vi "CtrExtTrigAuger.vi"() -> ()   [LabVIEW 2014]
uses:
  FPGA state.ctl
  <vilib>/Platform/TimedLoop/XDataNode/timing_clust.ctl
  <vilib>/Platform/TimedLoop/XDataNode/nitl_modes.ctl
  <vilib>/Platform/TimedLoop/XDataNode/wakeup.ctl
  <vilib>/rvi/Emulation/niFpgaSctlEmulationGetInTimedLoop.vi
  <vilib>/rvi/Emulation/niFpgaEmulationReportErrorSimple.vi
  <vilib>/rvi/Emulation/niFpgaGetClockAttributes.vi
  <vilib>/rvi/Emulation/niFpgaCriticalErrorInLSC.vi
  <vilib>/rvi/eio/common/nirviEmuTemplateMethod_errors.vi
  <vilib>/rvi/Emulation/niFpgaProcessEmulError.vi
  <vilib>/rvi/interface/RandomDataEmulation/niFpgaRandomDataHandleErrors.vi
  <vilib>/Platform/TimedLoop/XDataNode/XDataNode.xnode
  <vilib>/eio/EIONode/EIONode.xnode
  <vilib>/rvi/DataTransferAndStorage/Container/XNode/niFpgaContainer.xnode
  <vilib>/rvi/interface/RandomDataEmulation/nirviRandomDataFpgaReadWriteTemplate.vi
  <vilib>/Platform/TimedLoop/XDataNode/XDNodeRunTimeDep.lvlib
panel:
  in  "Sample Count":u32
  in  "Sample Period":u32
  out "Overflow":bool
  in  "Trigger Mode":T1(ring)
  # "Acquisition can be controlled by external trigger\n(through PXI backplane or input connector)\nor by the FPGA 25 MHz Clock."
  # "ExtTrig AugerCounter"
  # "Each U64 FIFO element is a pair of U32 with\n28 bits data, 4 bit ID in most significant bits\nID 0-7 for data channels, 8 for clock and 9 for trig count\n\nOn trigger return sample count, delta T in first element,\nand counts since last trigger on the eight data channels\n(7 for Auger plus aux) in the next 4 elements\n\nOn overflow, set trigger mode to off and flush FIFO\nOFF mode clears overflow, also resests sample count"
  # "(40 ns/25 MHz)"
  # "(0 for free-run)"
  # "FPGA DMA-FIFO CANNOT be cleared by FPGA,\nonly by PC Host VI. Ctr Overflow will be on when\nFPGA-side FIFO is full!"
  # "Red for overflow\ngreen for normal"
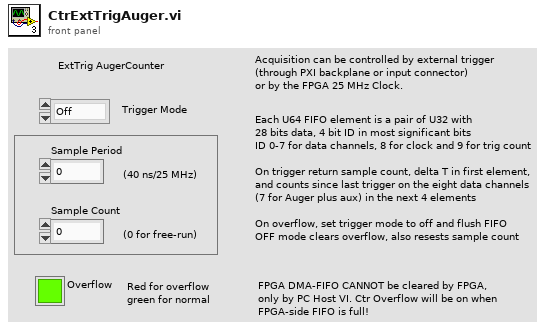
[diagram p1: front panel]
types:
  T1 = enum8{"Off", "PXI Trig0", "DIO-08 Trig", "Int Timer"}
  T2 = typedef "FPGA state.ctl" = enum8{"Wait", "Triggered", "Transfer 1", "Transfer 2", "Transfer 3", "Transfer 4", "Overflow"}
  T3 = typedef "XDNodeRunTimeDep.lvlib/timing_clust.ctl" = cluster{"Expected End [f-1]":u64, "Actual End [f-1]":u64, "Finished Late? [f-1]":bool, "Expected End [i-1]":u64, "Actual End [i-1]":u64, "Finished Late? [i-1]":bool, "Expected Start [i]":u64, "Actual Start [i]":u64, "Expected Start [f]":u64, "Actual Start [f]":u64, "Source Name":string, "Structure Name":string, "Period":i64, "Deadline":i64, "Offset":i64, "Start":i64, "Priority":i32, "Timeout":i32, "Mode":T4, "Wakeup Reason":T5, "Error":errorcluster, "Source Type":string, "Secondary Source Type":string, "Global End Time":u64, "Global Start Time":u64, "Frame Duration":u64, "Iteration Duration":u64, "Assigned CPU":i32, "I/O Scan Engine Mode":u32}
  T4 = typedef "XDNodeRunTimeDep.lvlib/nitl_modes.ctl" = enum32{"No Change", "Process missed periods, maintain original phase", "Discard missed periods, maintain original phase", "Process missed periods, ignore original phase", "Discard missed periods, ignore original phase"}
  T5 = typedef "XDNodeRunTimeDep.lvlib/wakeup.ctl" = enum32{"Normal", "Aborted", "Asynchronous wakeup", "Timing source error", "Timed loop error", "Timeout"}
  T6 = enum8{"Off", "PXI Trig0", "DIO-08 Trig", "Clocked"}
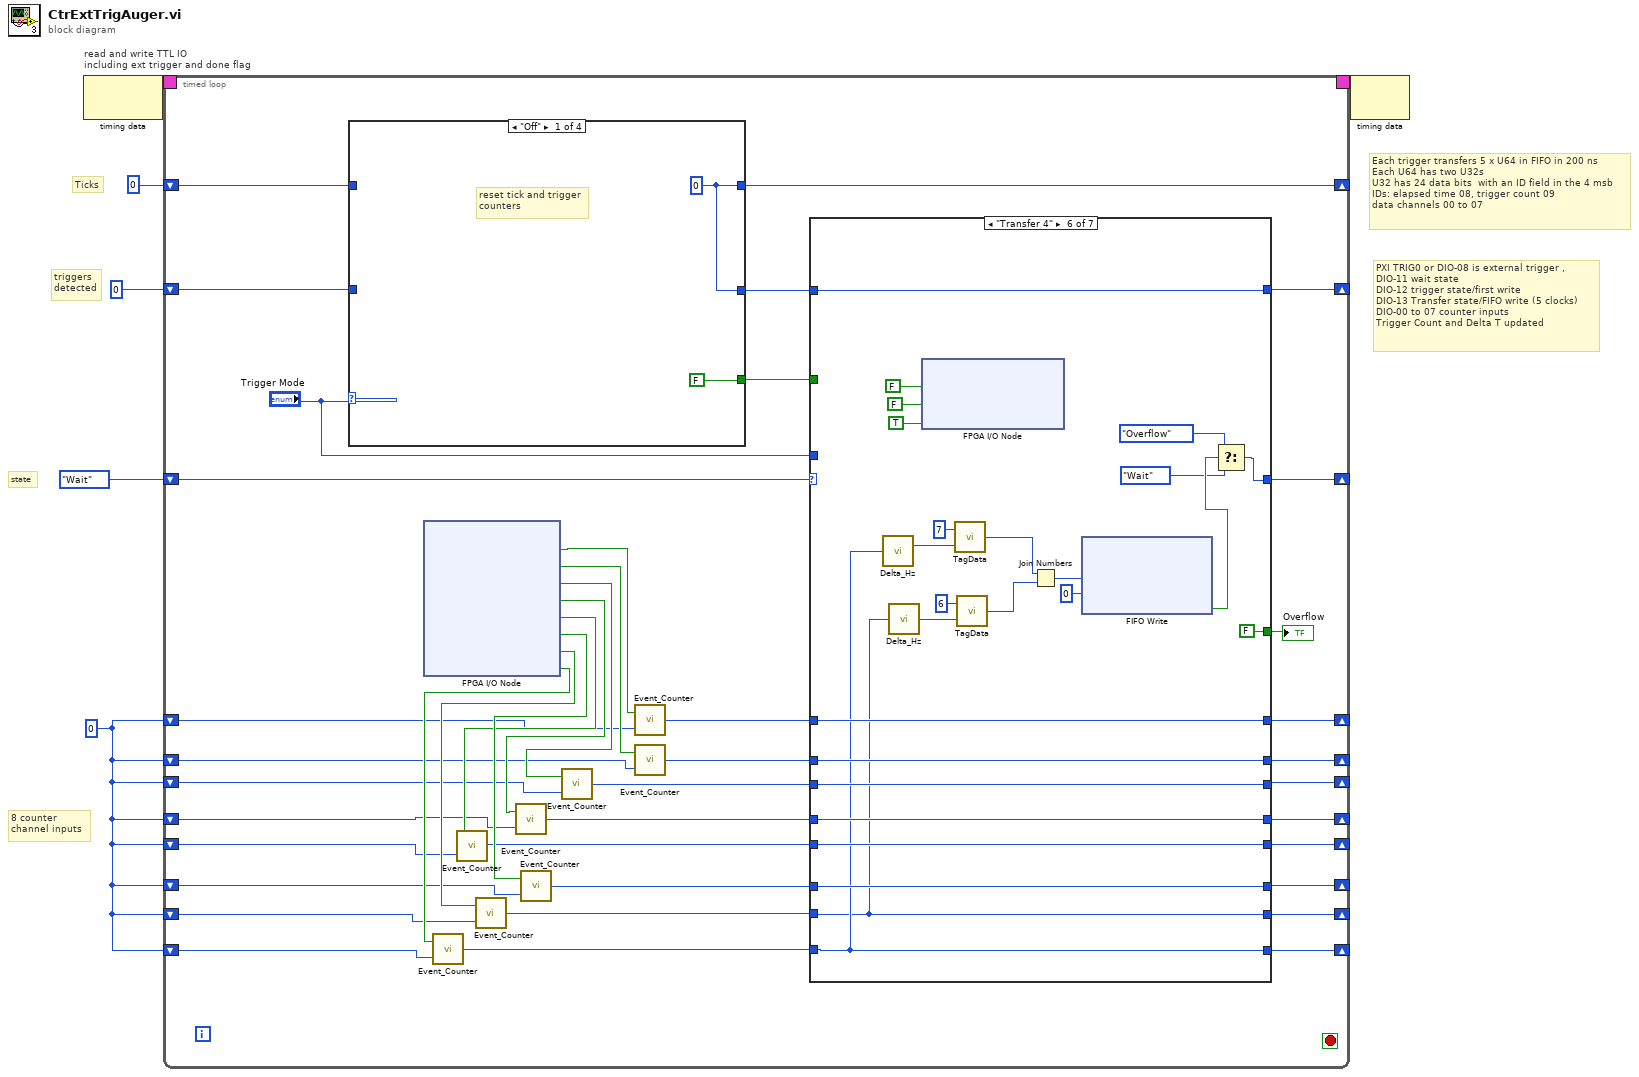
[diagram p0: block diagram]
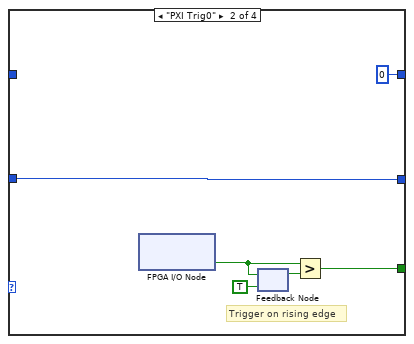
[diagram p2: hidden frame]
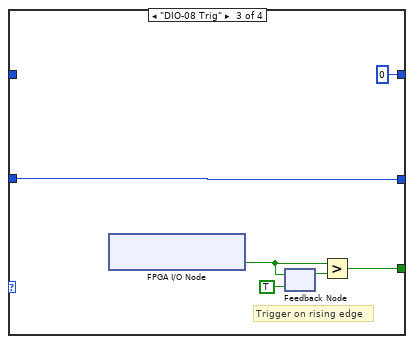
[diagram p3: hidden frame]
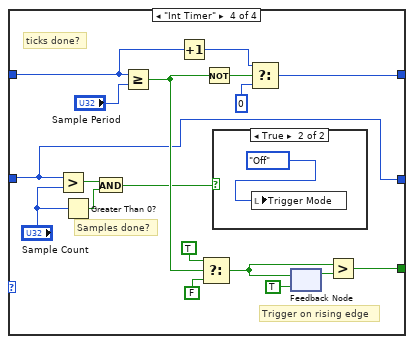
[diagram p4: hidden frame]
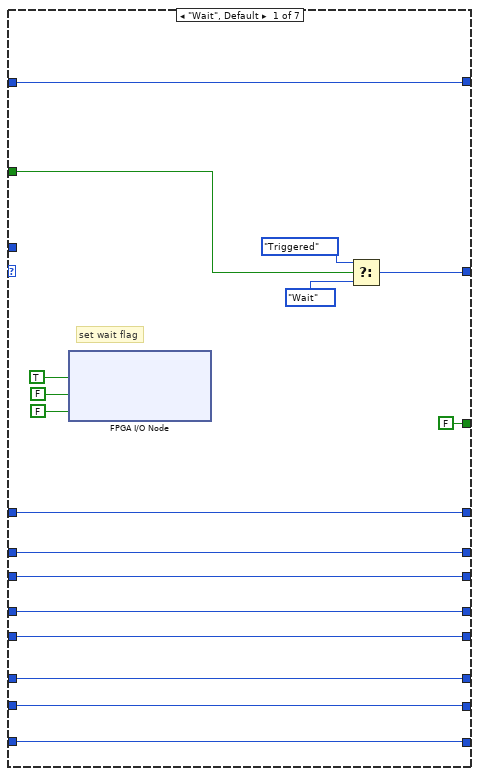
[diagram p6: hidden frame]
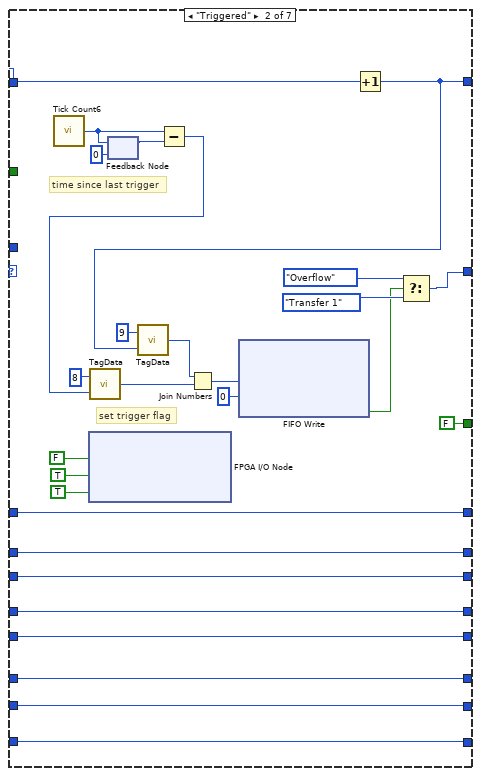
[diagram p7: hidden frame]
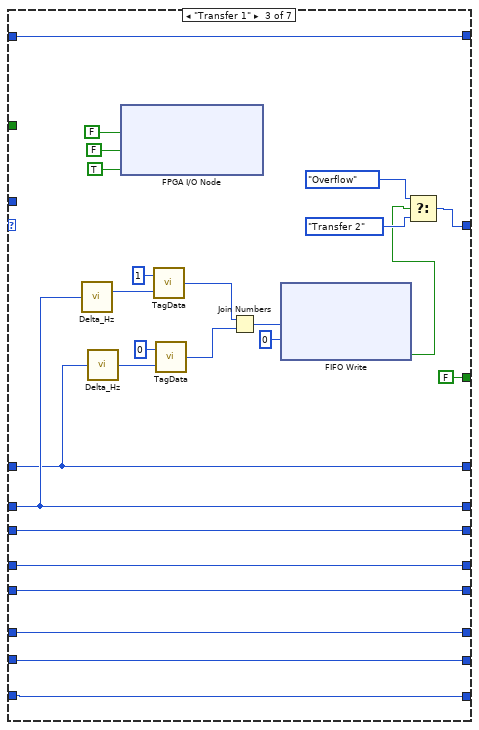
[diagram p8: hidden frame]
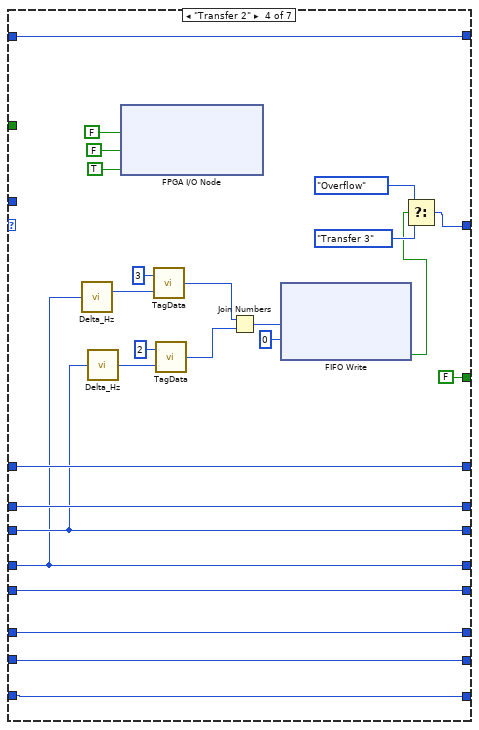
[diagram p9: hidden frame]
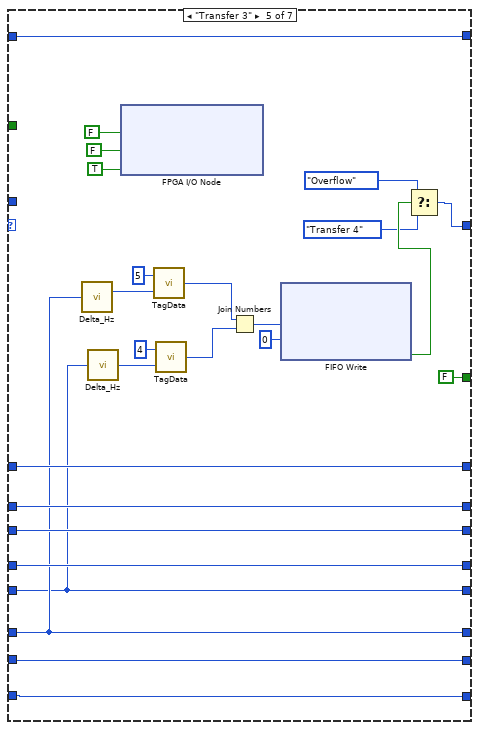
[diagram p10: hidden frame]
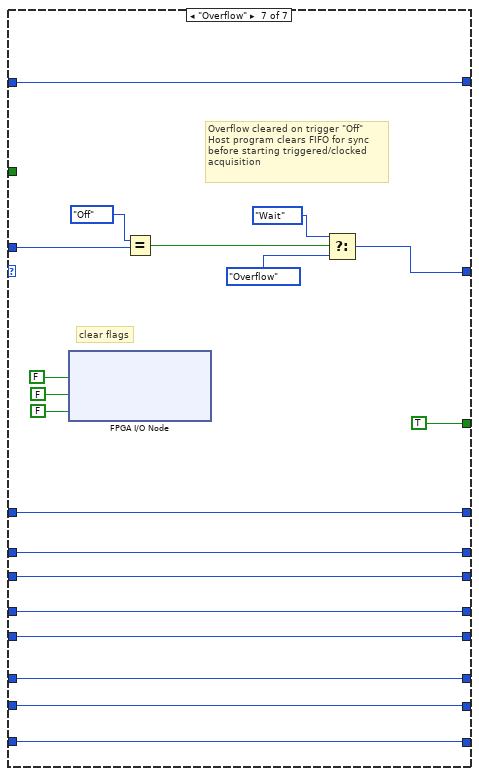
[diagram p11: hidden frame]
diagram:
  w1 = u32 0 ("Counts out")
  # "Each trigger transfers 5 x U64 in FIFO in 200 ns\nEach U64 has two U32s\nU32 has 24 data bits  with an ID field in the 4 msb\nIDs: elapsed time 08, trigger count 09\ndata channels 00 to 07"
  # "8 counter\nchannel inputs"
  # "Ticks"
  # "state"
  # "triggers\ndetected"
  # "PXI TRIG0 or DIO-08 is external trigger ,\nDIO-11 wait state\nDIO-12 trigger state/first write \nDIO-13 Transfer state/FIFO write (5 clocks)\nDIO-00 to 07 counter inputs \nTrigger Count and Delta T updated"
  n1 = node-c288() -> (w6:T3)  [unwired: 1 in]
  n2 = timed-loop "read and write TTL IO\nincluding ext trigger and done flag" {
    timing: w6 -> [_]
    timing-out: [_] -> w5
    shift-right: [w47] -> _
    shift-left: FPGA_state."Wait" -> [w48]
    shift-right: [w46] -> _
    shift-left: u32 0 -> [w12]
    shift-right: [w8] -> _
    shift-left: u32 0 -> [w9]
    shift-right: [w14] -> _
    shift-left: w1 -> [w30]
    shift-right: [w17] -> _
    shift-left: w1 -> [w31]
    shift-right: [w16] -> _
    shift-left: w1 -> [w35]
    shift-right: [w20] -> _
    shift-left: w1 -> [w36]
    shift-right: [w23] -> _
    shift-left: w1 -> [w39]
    shift-right: [w24] -> _
    shift-left: w1 -> [w38]
    shift-right: [w27] -> _
    shift-left: w1 -> [w40]
    shift-right: [w28] -> _
    shift-left: w1 -> [w41]
    stop <- _ stop-if-true
    n3 = case shown="\"Off\"" "Trigger Mode" {
      tunnel: [FALSE ("Connector0/DIO8") w52 w59 w78] -> w10
      tunnel: w12 -> [_ w56 w62 w63]
      tunnel: [w49 w56 w62 w63] -> w11
      tunnel: w9 -> [_ _ _ w68]
      tunnel: [w49 u32 0 u32 0 w73] -> w8
      frame "Off" {
        w49 = u32 0
        # "reset tick and trigger\ncounters"
      }
      frame "PXI Trig0" {
        # "Trigger on rising edge"
        n4 = xnode "FPGA I/O Node"() -> ("TRIG0"=w53:bool)  [unwired: 1 in, 1 out]
        n5 = feedback #1(TRUE ("set")) -> (w54:bool)
        n6 = feedback-in #1(w53) -> ()
        n7 = Greater?(x=w53, y=w54) -> (0:w52:bool)
      }
      frame "DIO-08 Trig" {
        # "Trigger on rising edge"
        n8 = xnode "FPGA I/O Node"() -> ("Connector0/DIO8"=w58:bool)  [unwired: 1 in, 1 out]
        n9 = feedback #2(TRUE ("set")) -> (w61:bool)
        n10 = feedback-in #2(w58) -> ()
        n11 = Greater?(x=w58, y=w61) -> (0:w59:bool)
      }
      frame "Int Timer" {
        # "ticks done?"
        # "Samples done?"
        # "Trigger on rising edge"
        n12 = Greater?(x=w63, y="Sample Count") -> (0:w65:bool)
        n13 = Greater Than 0?(x="Sample Count") -> (x > 0?=w67:bool)
        n14 = And(x=w65, y=w67) -> (x .and. y?=w64:bool)
        n15 = Greater Or Equal?(x=w68, y="Sample Period") -> (x >= y?=w72:bool)
        n16 = Increment(x=w68) -> (x+1=w71:u32)
        n17 = Select(t=TRUE, s=w72, f=FALSE) -> (s? t:f=w74:bool)
        n18 = Not(x=w72) -> (.not. x?=w70:bool)
        n19 = case shown="True" w64 {
          frame False {
          }
          frame True {
            n20 = local write "Trigger Mode"(T1."Off" ("Trigger Mode")) -> ()
          }
        }
        n21 = Select(t=w71, s=w70, f=u32 0) -> (s? t:f=w73:u32)
        n22 = feedback #3(TRUE ("set")) -> (w80:bool)
        n23 = feedback-in #3(w74) -> ()
        n24 = Greater?(x=w74, y=w80) -> (0:w78:bool)
      }
    }
    n25 = xnode "FPGA I/O Node"() -> ("Connector0/DIO0"=w32:bool, "Connector0/DIO1"=w33:bool, "Connector0/DIO2"=w34:bool, "Connector0/DIO3"=w37:bool, "Connector0/DIO4"=w42:bool, "Connector0/DIO5"=w43:bool, "Connector0/DIO6"=w44:bool, "Connector0/DIO7"=w45:bool)  [unwired: 8 in, 8 out]
    n26 = call "Event_Counter.vi"("Counts in"=w41, "input"=w45) -> ("Counts out"=w29:u32)
    n27 = call "Event_Counter.vi"("Counts in"=w39, "input"=w42) -> ("Counts out"=w22:u32)
    n28 = call "Event_Counter.vi"("Counts in"=w40, "input"=w44) -> ("Counts out"=w26:u32)
    n29 = call "Event_Counter.vi"("Counts in"=w36, "input"=w37) -> ("Counts out"=w21:u32)
    n30 = call "Event_Counter.vi"("Counts in"=w38, "input"=w43) -> ("Counts out"=w25:u32)
    n31 = call "Event_Counter.vi"("Counts in"=w35, "input"=w34) -> ("Counts out"=w19:u32)
    n32 = call "Event_Counter.vi"("Counts in"=w30, "input"=w32) -> ("Counts out"=w15:u32)
    n33 = call "Event_Counter.vi"("Counts in"=w31, "input"=w33) -> ("Counts out"=w18:u32)
    n34 = case shown="\"Transfer 4\"" w48 {
      tunnel: [w96 w104 w128 w153 w178 w203 w227] -> w47
      tunnel: w11 -> [w94 w126 w144 w169 w194 w219 w245]
      tunnel: [w94 w105 w144 w169 w194 w219 w245] -> w46
      tunnel: w10 -> [w95 _ _ _ _ _ _]
      tunnel: w29 -> [w93 w119 w137 w163 w190 w208 w244]
      tunnel: [w93 w119 w137 w163 w190 w208 w244] -> w28
      tunnel: [w92 w118 w138 w164 w191 w207 w243] -> w27
      tunnel: w26 -> [w92 w118 w138 w164 w191 w207 w243]
      tunnel: w25 -> [w91 w117 w139 w165 w183 w210 w242]
      tunnel: [w91 w117 w139 w165 w183 w210 w242] -> w24
      tunnel: [w90 w116 w140 w166 w182 w209 w241] -> w23
      tunnel: w22 -> [w90 w116 w140 w166 w182 w209 w241]
      tunnel: w21 -> [w89 w112 w136 w157 w184 w211 w240]
      tunnel: [w89 w112 w136 w157 w184 w211 w240] -> w20
      tunnel: w19 -> [w87 w115 w141 w158 w185 w212 w238]
      tunnel: w18 -> [w88 w114 w133 w160 w187 w214 w239]
      tunnel: [w88 w114 w133 w160 w187 w214 w239] -> w17
      tunnel: [w87 w115 w141 w158 w185 w212 w238] -> w16
      tunnel: w15 -> [w86 w113 w132 w159 w186 w213 w237]
      tunnel: [w86 w113 w132 w159 w186 w213 w237] -> w14
      tunnel: [FALSE ("Connector0/DIO11") FALSE ("Connector0/DIO11") FALSE ("Connector0/DIO11") FALSE ("Connector0/DIO11") FALSE ("Connector0/DIO11") FALSE ("Connector0/DIO11") TRUE ("Connector0/DIO11")] -> w13
      tunnel: "Trigger Mode" -> [_ _ _ _ _ _ w232]
      frame "Wait", Default {
        # "set wait flag"
        n35 = xnode "FPGA I/O Node"("Connector0/DIO11"=TRUE, "Connector0/DIO12"=FALSE ("Connector0/DIO11"), "Connector0/DIO13"=FALSE ("Connector0/DIO11")) -> ()  [unwired: 3 in, 3 out]
        n36 = Select(t=FPGA_state."Triggered", s=w95, f=FPGA_state."Wait") -> (s? t:f=w96:T2)
      }
      frame "Triggered" {
        # "time since last trigger"
        # "set trigger flag"
        n37 = Increment(x=w126) -> ()  [unwired: 1 out]
        n38 = call "Tick Count6"() -> ("Tick Count(Ticks)"=w124:u32)
        n39 = xnode "FPGA I/O Node"("Connector0/DIO11"=FALSE, "Connector0/DIO12"=TRUE ("Connector0/DIO11"), "Connector0/DIO13"=TRUE ("Connector0/DIO11")) -> ()  [unwired: 3 in, 3 out]
        n40 = feedback-in #4(w124) -> ()
        n41 = feedback #4(u32 0 ("Tick Count(Ticks)")) -> (w125:u32)
        n42 = Subtract(x=w124, y=w125) -> (x-y=w99:u32)
        n43 = call "TagData.vi"("Data"=w99, "Tag"=u8 8) -> ("Data 2"=w106:u32)
        n44 = Increment(x=w126) -> (x+1=w105:u32)
        n45 = call "TagData.vi"("Data"=w105, "Tag"=u8 9) -> ("Data 2"=w109:u32)
        n46 = Join Numbers(hi=w109, lo=w106) -> ((hi.lo)=w111:u64)
        n47 = xnode ("FIFO Write")("Element"=w111, "Timeout"=0) -> ("Timed Out?"=w101:bool)  [unwired: 1 in, 1 out]
        n48 = Select(t=FPGA_state."Overflow", s=w101, f=FPGA_state."Transfer 1") -> (s? t:f=w104:T2)
      }
      frame "Transfer 1" {
        n49 = call "Delta_Hz.vi"("Counts"=w133) -> ("Delta"=w134:u32)
        n50 = call "Delta_Hz.vi"("Counts"=w132) -> ("Delta"=w135:u32)
        n51 = xnode "FPGA I/O Node"("Connector0/DIO11"=FALSE ("Connector0/DIO15"), "Connector0/DIO12"=FALSE ("Connector0/DIO15"), "Connector0/DIO13"=TRUE ("Connector0/DIO15")) -> ()  [unwired: 3 in, 3 out]
        n52 = call "TagData.vi"("Data"=w134, "Tag"=u8 1) -> ("Data 2"=w146:u32)
        n53 = call "TagData.vi"("Data"=w135, "Tag"=u8 0) -> ("Data 2"=w142:u32)
        n54 = Join Numbers(hi=w146, lo=w142) -> ((hi.lo)=w151:u64)
        n55 = xnode ("FIFO Write")("Element"=w151, "Timeout"=0) -> ("Timed Out?"=w129:bool)  [unwired: 1 in, 1 out]
        n56 = Select(t=FPGA_state."Overflow", s=w129, f=FPGA_state."Transfer 2") -> (s? t:f=w128:T2)
      }
      frame "Transfer 2" {
        n57 = call "Delta_Hz.vi"("Counts"=w157) -> ("Delta"=w161:u32)
        n58 = call "Delta_Hz.vi"("Counts"=w158) -> ("Delta"=w162:u32)
        n59 = xnode "FPGA I/O Node"("Connector0/DIO11"=FALSE ("Connector0/DIO15"), "Connector0/DIO12"=FALSE ("Connector0/DIO15"), "Connector0/DIO13"=TRUE ("Connector0/DIO15")) -> ()  [unwired: 3 in, 3 out]
        n60 = call "TagData.vi"("Data"=w161, "Tag"=u8 3) -> ("Data 2"=w171:u32)
        n61 = call "TagData.vi"("Data"=w162, "Tag"=u8 2) -> ("Data 2"=w167:u32)
        n62 = Join Numbers(hi=w171, lo=w167) -> ((hi.lo)=w176:u64)
        n63 = xnode ("FIFO Write")("Element"=w176, "Timeout"=0) -> ("Timed Out?"=w155:bool)  [unwired: 1 in, 1 out]
        n64 = Select(t=FPGA_state."Overflow", s=w155, f=FPGA_state."Transfer 3") -> (s? t:f=w153:T2)
      }
      frame "Transfer 3" {
        n65 = call "Delta_Hz.vi"("Counts"=w183) -> ("Delta"=w188:u32)
        n66 = call "Delta_Hz.vi"("Counts"=w182) -> ("Delta"=w189:u32)
        n67 = xnode "FPGA I/O Node"("Connector0/DIO11"=FALSE ("Connector0/DIO15"), "Connector0/DIO12"=FALSE ("Connector0/DIO15"), "Connector0/DIO13"=TRUE ("Connector0/DIO15")) -> ()  [unwired: 3 in, 3 out]
        n68 = call "TagData.vi"("Data"=w188, "Tag"=u8 5) -> ("Data 2"=w196:u32)
        n69 = call "TagData.vi"("Data"=w189, "Tag"=u8 4) -> ("Data 2"=w192:u32)
        n70 = Join Numbers(hi=w196, lo=w192) -> ((hi.lo)=w201:u64)
        n71 = xnode ("FIFO Write")("Element"=w201, "Timeout"=0) -> ("Timed Out?"=w181:bool)  [unwired: 1 in, 1 out]
        n72 = Select(t=FPGA_state."Overflow", s=w181, f=FPGA_state."Transfer 4") -> (s? t:f=w178:T2)
      }
      frame "Transfer 4" {
        n73 = call "Delta_Hz.vi"("Counts"=w208) -> ("Delta"=w215:u32)
        n74 = call "Delta_Hz.vi"("Counts"=w207) -> ("Delta"=w216:u32)
        n75 = xnode "FPGA I/O Node"("Connector0/DIO11"=FALSE ("Connector0/DIO15"), "Connector0/DIO12"=FALSE ("Connector0/DIO15"), "Connector0/DIO13"=TRUE ("Connector0/DIO15")) -> ()  [unwired: 3 in, 3 out]
        n76 = call "TagData.vi"("Data"=w215, "Tag"=u8 7) -> ("Data 2"=w221:u32)
        n77 = call "TagData.vi"("Data"=w216, "Tag"=u8 6) -> ("Data 2"=w217:u32)
        n78 = Join Numbers(hi=w221, lo=w217) -> ((hi.lo)=w226:u64)
        n79 = xnode ("FIFO Write")("Element"=w226, "Timeout"=0) -> ("Timed Out?"=w206:bool)  [unwired: 1 in, 1 out]
        n80 = Select(t=FPGA_state."Overflow", s=w206, f=FPGA_state."Wait") -> (s? t:f=w203:T2)
      }
      frame "Overflow" {
        # "Overflow cleared on trigger \"Off\"\nHost program clears FIFO for sync\nbefore starting triggered/clocked\nacquisition"
        # "clear flags"
        n81 = xnode "FPGA I/O Node"("Connector0/DIO11"=FALSE, "Connector0/DIO12"=FALSE ("Connector0/DIO11"), "Connector0/DIO13"=FALSE ("Connector0/DIO11")) -> ()  [unwired: 3 in, 3 out]
        n82 = Equal?(x=T6."Off" ("Trigger Mode"), y=w232) -> (x = y?=w230:bool)
        n83 = Select(t=FPGA_state."Wait", s=w230, f=FPGA_state."Overflow") -> (s? t:f=w227:T2)
      }
    }
    "Overflow" <- w13
  }
  n84 = node-c288(w5) -> ()  [unwired: 1 out]
